vi "Multi_OUI_NON.vi"(8 "errin":errorcluster caption="entrée d'erreur (pas d'erreur)", 9 "errinb":bool, 10 "Tableau":string[](array[string])) -> (0 "errout":errorcluster caption="sortie d'erreur", 3 "isok?":bool)   [LabVIEW 2020]
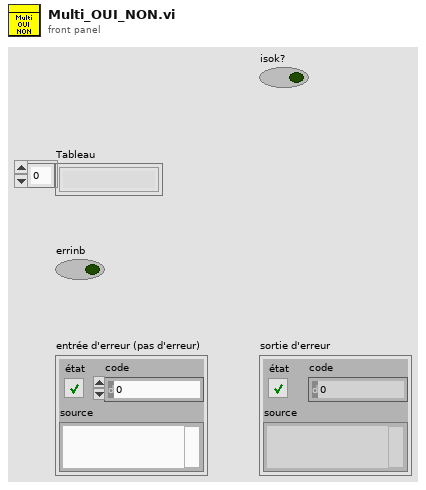
[diagram p1: front panel]
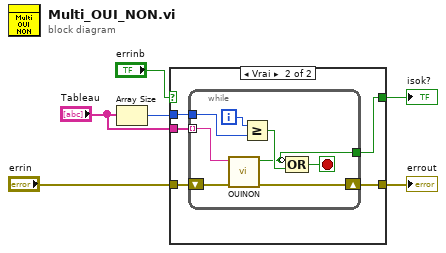
[diagram p0: block diagram]
diagram:
  n1 = Array Size(array="Tableau") -> (size(s)=w1:i32)
  n2 = case shown="Vrai" "errinb" {
    selector: "errinb" -> [w7 _]
    tunnel: "Tableau" -> [_ w13]
    tunnel: w1 -> [_ w12]
    tunnel: [w7 w11] -> w3
    tunnel: [w8 w10] -> w4
    tunnel: "errin" -> [w8 w9]
    frame False {
    }
    frame True {
      n3 = while {
        tunnel: w13 -> [w19] mode=indexing
        tunnel: w12 -> [w20]
        shift-right: [w17] -> w10
        shift-left: w9 -> [w18]
        tunnel: [w14] -> w11
        i -> [w21]
        stop <- w15 stop-if-true
        n4 = call "OUINON.vi"("errin"=w18, "image"=w19) -> ("error out"=w17:errorcluster, "OUI/NON"=w14:bool)  [unwired: 8 in]
        n5 = Greater Or Equal?(x=w21, y=w20) -> (x >= y?=w16:bool)
        n6 = Compound Arithmetic op=OR ("Opérateur arithmétique")(invert w14, w16) -> (w15:bool)
      }
    }
  }
  "errout" <- w4
  "isok?" <- w3
